vi "Perform Action.vi"(8 "error in":errorcluster, 10 "Input":variant, 11 "Virt Instr Base in":refnum<class "Virtual Instrument.lvclass">) -> (0 "error out":errorcluster, 2 "Output":variant, 3 "Virt Instr Base out":refnum<class "Virtual Instrument.lvclass">)   [LabVIEW 2023, in "HAL.lvlib" / "Virtual Instrument.lvclass"]
uses:
  Virtual Instrument.lvclass
  Virtual Instrument.lvclass/Virtual Instrument.ctl
  Perform Action Strategy/Perform Action Strategy.lvclass
  Scaling Strategy/Scaling Strategy.lvclass
  Instrument/Instrument.lvclass
  D:/git/HAL/HAL/Instrument/Instrument.lvclass
  D:/git/HAL/HAL/Interfaces/IPerform Action/IPerform Action.lvclass
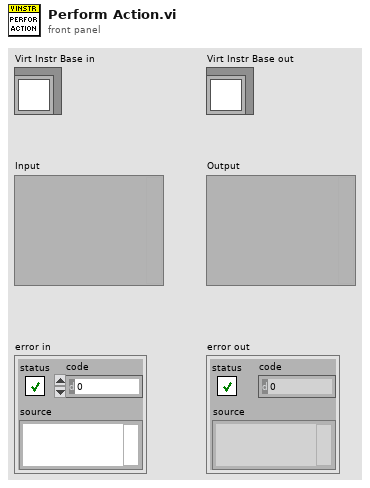
[diagram p1: front panel]
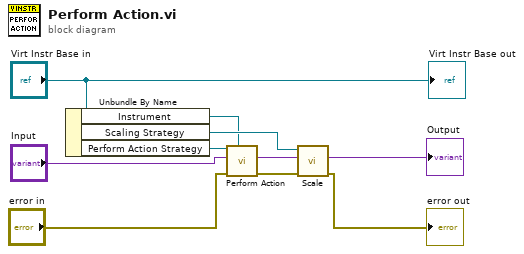
[diagram p0: block diagram]
diagram:
  n1 = Unbundle By Name("Virt Instr Base in") -> ("Instrument"=w1:refnum<class "Instrument.lvclass">, "Scaling Strategy"=w6:refnum<class "Scaling Strategy.lvclass">, "Perform Action Strategy"=w9:refnum<class "Perform Action Strategy.lvclass">)
  n2 = call-dynamic "Perform Action.vi"("IPerform Action"=w1, "error in"="error in", "Input"="Input", "Perform Action Strategy in"=w9) -> ("error out"=w4:errorcluster, "Output"=w5:variant)  [unwired: 5 in, 1 out]
  n3 = call-dynamic "Scale.vi"("error in"=w4, "Input"=w5, "Scaling Strategy in"=w6) -> ("error out"=→"error out":errorcluster, "Output"=→"Output":variant)  [unwired: 6 in, 1 out]
  "Virt Instr Base out" <- "Virt Instr Base in"
